vi "Add Meas Plugin Controls - Multiple Converter.vi"(11 "error in":errorcluster) -> (15 "error out":errorcluster)   [LabVIEW 2021, in "Converter.lvlib"]
uses:
  Converter.lvlib
  Converter Reusables/Converter Reusables.lvlib
  Path Functions/Path Functions.lvlib
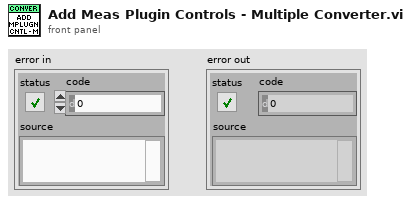
[diagram p1: front panel]
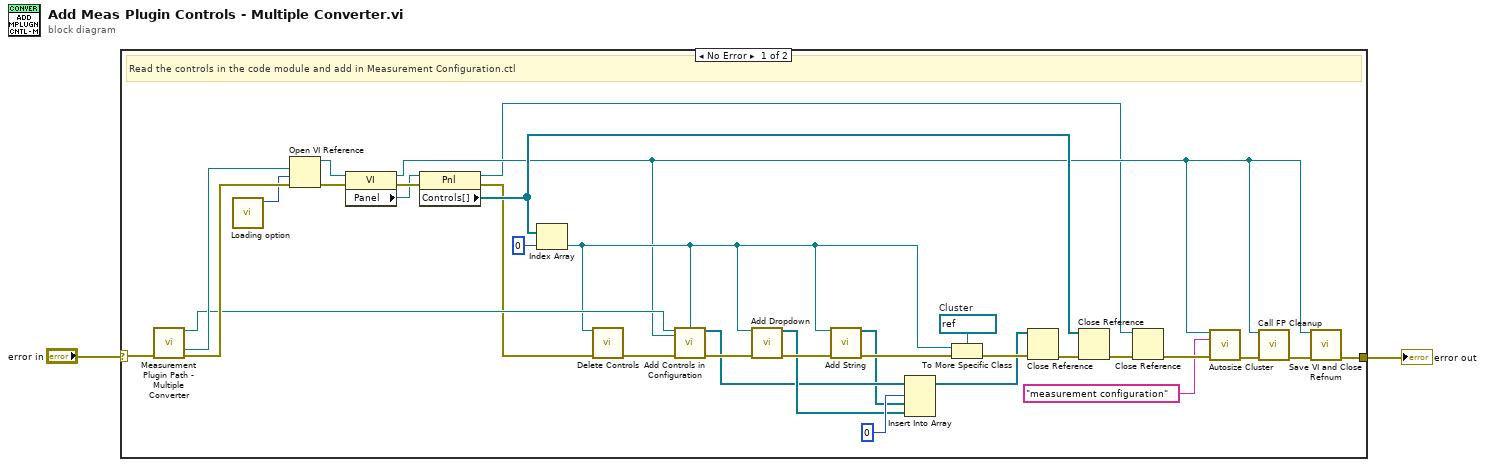
[diagram p0: block diagram]
diagram:
  n1 = case shown="No Error" "error in" {
    selector: "error in" -> [w24 w36]
    tunnel: [w30 w36] -> w2
    frame No Error {
      w29 = refnum<vi> refnum  # Cluster
      # "Read the controls in the code module and add in Measurement Configuration.ctl"
      n2 = call "Measurement Plugin Path - Multiple Converter.vi"("error in"=w24) -> ("new code module"=w17:path, "input controls"=w23:path, "error out"=w25:errorcluster)  [unwired: 2 in, 10 out]
      n3 = call "Loading option.vi"() -> ("options"=w3:i32)  [unwired: 11 in]
      n4 = Open VI Reference(vi path=w23, options=w3, error in (no error)=w25) -> (vi reference=w7:refnum<vi>, error out=w31:errorcluster)  [unwired: 3 in]
      n5 = property class="VI"(reference=w7, error in=w31) -> (reference out=w6:refnum<vi>, error out=w35:errorcluster, "Panel"=w5:refnum<vi>)
      n6 = property class="Pnl"(reference=w5, error in=w35) -> (reference out=w4:refnum<vi>, error out=w15:errorcluster, "Controls[]"=w21:refnum<vi>[])
      n7 = Index Array(array=w21, index=0) -> (element=w14:refnum<vi>)
      n8 = call "Delete Controls.vi"("control in"=w14, "error in"=w15) -> ("error out"=w16:errorcluster)  [unwired: 13 in]
      n9 = call "Add Controls in Configuration.vi"("new code module"=w17, "vi reference"=w6, "configuration ctl refnum"=w14, "error in"=w16) -> ("controls reference"=w10:refnum<vi>[], "error out"=w18:errorcluster)  [unwired: 10 in]
      n10 = call "Add Dropdown.vi"("control ref"=w14, "error in"=w18) -> ("combo box ref"=w11:refnum<vi>[], "error out"=w12:errorcluster)  [unwired: 12 in]
      n11 = call "Add String.vi"("control ref"=w14, "error in"=w12) -> ("string ref"=w8:refnum<vi>[], "error out"=w13:errorcluster)  [unwired: 12 in]
      n12 = Insert Into Array(array=w10, index=0, new element #1=w8, new element #2=w11) -> (w9:refnum<vi>[])
      n13 = To More Specific Class(target class=w29, reference=w14, error in=w13) -> (error out=w27:errorcluster)  [unwired: 1 out]
      n14 = Close Reference(reference=w9, error in (no error)=w27) -> (error out=w20:errorcluster)
      n15 = Close Reference(reference=w21, error in (no error)=w20) -> (error out=w19:errorcluster)
      n16 = Close Reference(reference=w4, error in (no error)=w19) -> (error out=w33:errorcluster)
      n17 = call "Autosize Cluster.vi"("vi refnum"=w6, "name"="measurement configuration" ("name/order"), "error in"=w33) -> ("error out"=w22:errorcluster)  [unwired: 12 in]
      n18 = call "Call FP Cleanup.vi"("vi"=w6, "error in"=w22) -> ("error out"=w26:errorcluster)  [unwired: 13 in]
      n19 = call "Save VI and Close Refnum.vi"("vi refnum"=w6, "error in"=w26) -> ("error out"=w30:errorcluster)  [unwired: 13 in]
    }
    frame Error {
    }
  }
  "error out" <- w2
